vi "OAT Even Time or Speed Segment (XY, 1D Array).vi"(0 "XY signals":cluster{"X":dbl[], "Y":dbl[]}[](array[cluster]) {"X" format="%.2f"; "Y" format="%.2f"}, 1 "x-axis selection":u16(ring)=2 items=["Time", "Revolution", "RPM"], 2 "reset? (F)":bool, 3 "phase input? (F)":bool, 5 "speed profile":T4 {"speed [RPM]" format="%.2f"; "time [s]" format="%.2f"}, 7 "position info":T2, 9 "pulse/revolution (1)":i32=1, 11 "error in (no error)":errorcluster, 12 "segment settings":cluster{"start":dbl, "end":dbl, "step size":dbl} {"step size" format="%.2f"; "end" min=0.0 format="%.2f"; "start" min=0.0 format="%.2f"}, 13 "view info":T1={"dB on? (F)"=FALSE, "unwrap phase? (T)"=TRUE, "unit in degree? (T)"=TRUE}) -> (4 "XY signals out":cluster{"X":dbl[], "Y":dbl[]}[](array[cluster]) {"X" format="%.2f"; "Y" format="%.2f"}, 8 "position info out":T2, 10 "end reached?":bool, 14 "actual segment settings":T3 {"actual step size" format="%.2f"; "actual end" min=0.0 format="%.2f"; "actual start" min=0.0 format="%.2f"}, 15 "error out":errorcluster)   [LabVIEW 2017, in "SoundVib_OAUtility.lvlib"]
doc: "Divides an input signal into even-time segments or even-speed intervals. The input signal of this VI can be an even-angle signal or an XY signal. When you use this VI to divide an XY signal, the XY signal can be only the output of the OAT Order Magnitude and Phase VI or OAT Overall Level Plot VI. Wire data to the <B>even-angle signal</B> input to determine the polymorphic instance to use or manually select the instance."
uses:
  <vilib>/addons/Sound and Vibration/Order Analysis/Utility/SoundVib_OAUtility.lvlib
  <vilib>/addons/Sound and Vibration/Order Analysis/Tach Process/SubVIs/speed profile.ctl
  <vilib>/addons/Sound and Vibration/Order Analysis/Misc/OAT Position Info.ctl
  <vilib>/addons/Sound and Vibration/Order Analysis/Tach Process/SoundVib_TachProcess.lvlib
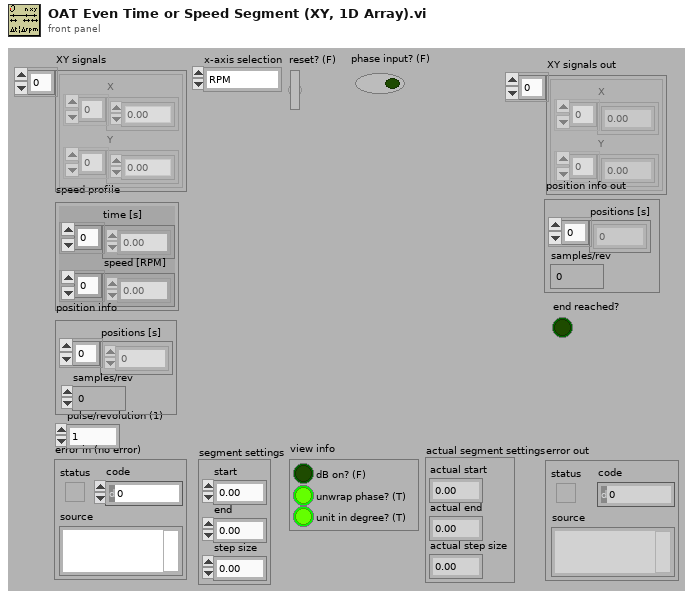
[diagram p1: front panel]
types:
  T1 = cluster{"dB on? (F)":bool, "unwrap phase? (T)":bool, "unit in degree? (T)":bool}
  T2 = typedef "OAT Position Info.ctl" = cluster{"positions [s]":dbl[], "samples/rev":dbl}
  T3 = cluster{"actual start":dbl, "actual end":dbl, "actual step size":dbl}
  T4 = typedef "SoundVib_TachProcess.lvlib/speed profile.ctl" = cluster{"time [s]":dbl[], "speed [RPM]":dbl[]}
  T5 = cluster{"last rev":dbl, "rev indice":dbl[], "time indice":dbl[], "RPM indice":dbl[]}
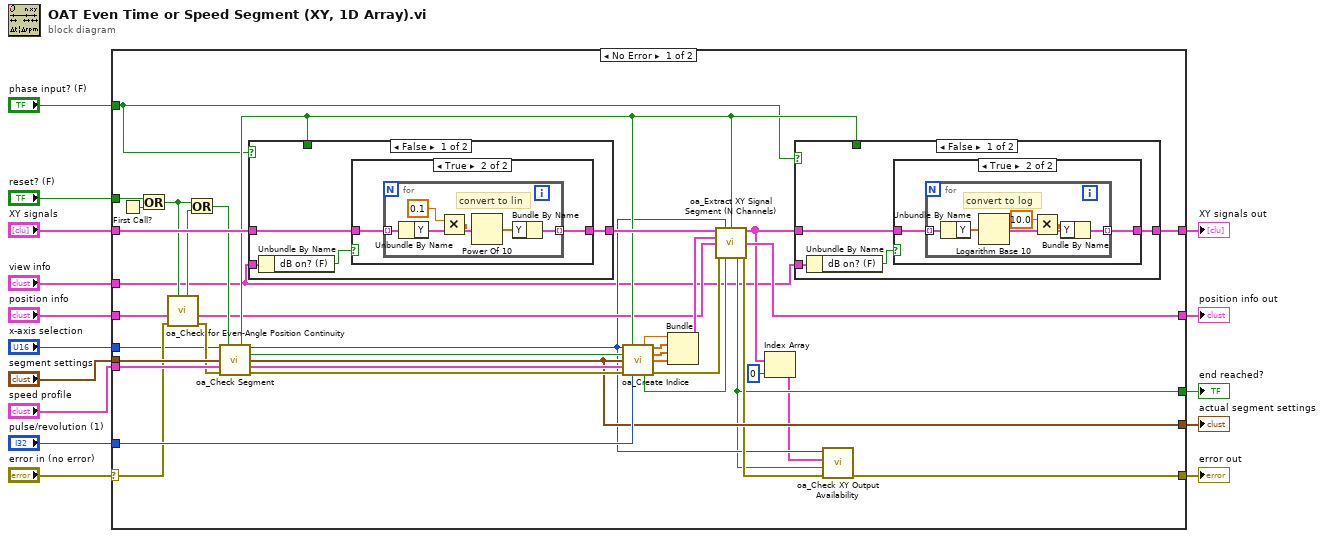
[diagram p0: block diagram]
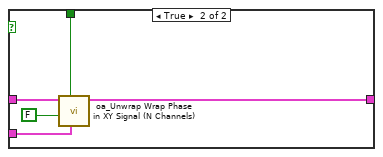
[diagram p3: hidden frame]
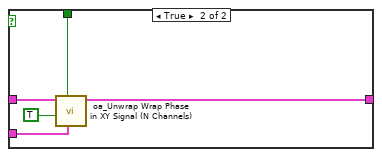
[diagram p5: hidden frame]
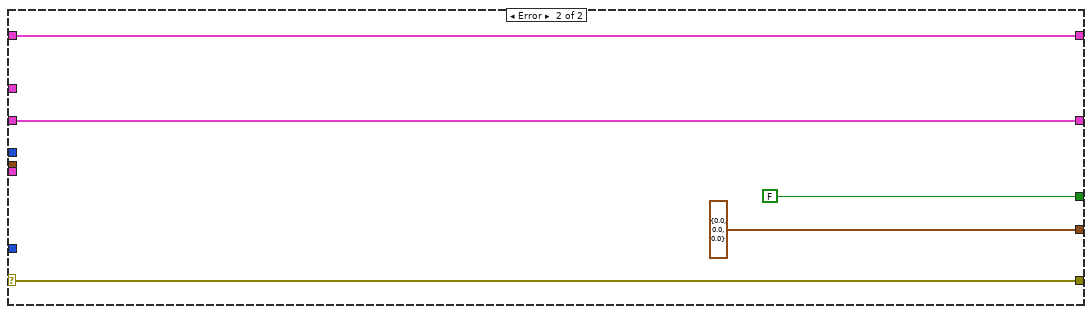
[diagram p6: hidden frame]
diagram:
  n1 = case shown="No Error" "error in (no error)" {
    selector: "error in (no error)" -> [w27 w94]
    tunnel: [w24 w94] -> w1
    tunnel: "reset? (F)" -> [w36 _]
    tunnel: "x-axis selection" -> [w23 _]
    tunnel: "segment settings" -> [w46 _]
    tunnel: "speed profile" -> [w31 _]
    tunnel: [w44 cluster{"start":dbl, "end":dbl, "step":dbl} {"start"=0.0, "end"=0.0, "step"=0.0} ("steps output")] -> w2
    tunnel: "pulse/revolution (1)" -> [w45 _]
    tunnel: "XY signals" -> [w39 w92]
    tunnel: [w21 FALSE ("finish?")] -> w4
    tunnel: "position info" -> [w42 w91]
    tunnel: [w37 w92] -> w5
    tunnel: [w40 w91] -> w3
    tunnel: "phase input? (F)" -> [w17 _]
    tunnel: "view info" -> [w16 _]
    frame No Error {
      n2 = First Call?() -> (First Call?: T/F=w35:bool)
      n3 = Or(x=w36, y=w35) -> (x .or. y?=w29:bool)
      n4 = call <vilib>:"oa_Check for Even-Angle Position Continuity.vi"("reset in"=w29, "error in (no error)"=w27, "even-angle position info"=w42) -> ("error out"=w26:errorcluster, "even-angle position info dup"=w30:T2, "position not continuous"=w28:bool)  [unwired: 6 in]
      n5 = Or(x=w29, y=w28) -> (x .or. y?=w32:bool)
      n6 = call <vilib>:"oa_Check Segment.vi"("X axis selection"=w23, "reset?(F)"=w32, "segment position"=w46, "speed profile"=w31, "error in (no error)"=w26) -> ("reset out"=w33:bool, "X axis selection"=w22:u16, "step found?"=w51:bool, "segment position out"=w44:cluster{"start":dbl, "end":dbl, "step size":dbl}, "dul speed profile"=w52:T4, "error out"=w53:errorcluster)  [unwired: 5 in]
      n7 = case shown="False" w17 {
        tunnel: w39 -> [w73 w89]
        tunnel: [w72 w88] -> w38
        tunnel: w33 -> [_ w87]
        tunnel: w16 -> [w75 w85]
        frame False {
          n8 = Unbundle By Name(w75) -> ("dB on? (F)"=w74:bool)
          n9 = case shown="True" w74 {
            tunnel: w73 -> [w76 w78]
            tunnel: [w76 w77] -> w72
            frame False {
            }
            frame True {
              n10 = for {
                tunnel: w78 -> [w83] mode=indexing
                tunnel: [w82] -> w77 mode=indexing
                # "convert to lin"
                n11 = Unbundle By Name(w83) -> ("Y"=w81:dbl[])
                n12 = Multiply(x=0.1 ("last rev"), y=w81) -> (x*y=w80:dbl[])
                n13 = Power Of 10(x=w80) -> (10^x=w84:dbl[])
                n14 = Bundle By Name(cluster=w83, "Y"=w84) -> (w82:cluster{"X":dbl[], "Y":dbl[]})
              }
            }
          }
        }
        frame True {
          n15 = call <vilib>:"oa_Unwrap Wrap Phase in XY Signal (N Channels).vi"("view"=w85, "reset? (F)"=w87, "Unwrap?"=TRUE, "XY signals"=w89) -> ("XY signals out"=w88:cluster{"X":dbl[], "Y":dbl[]}[])  [unwired: 7 in]
        }
      }
      n16 = call <vilib>:"oa_Create Indice.vi"("X axis selection"=w22, "reset?(F)"=w33, "step found?(F)"=w51, "steps input"=w44, "speed profile"=w52, "error in (no error)"=w53, "pulse/revolution (1)"=w45) -> ("last rev"=w47:dbl, "rev indice"=w48:dbl[], "time indice"=w49:dbl[], "RPM indice"=w50:dbl[], "reach end?"=w34:bool, "error out"=w41:errorcluster)  [unwired: 2 in, 1 out]
      n17 = Bundle("last rev"=w47, "rev indice"=w48, "time indice"=w49, "RPM indice"=w50) -> (w43:T5)  [unwired: 1 in]
      n18 = call <vilib>:"oa_Extract XY Signal Segment (N Channels).vi"("XY signals"=w38, "X axis selection"=w22, "reset? (F)"=w33, "trigger indices"=w43, "position info in"=w30, "error in (no error)"=w41, "indices end?"=w34) -> ("XY signals out"=w20:cluster{"X":dbl[], "Y":dbl[]}[], "position info out"=w40:T2, "reached end?"=w21:bool, "error out"=w25:errorcluster)  [unwired: 5 in]
      n19 = Index Array(array=w20, index=0) -> (element=w19:cluster{"X":dbl[], "Y":dbl[]})
      n20 = case shown="False" w17 {
        tunnel: w20 -> [w55 w71]
        tunnel: [w56 w70] -> w37
        tunnel: w16 -> [w57 w69]
        tunnel: w33 -> [_ w67]
        frame False {
          n21 = Unbundle By Name(w57) -> ("dB on? (F)"=w54:bool)
          n22 = case shown="True" w54 {
            tunnel: w55 -> [w58 w60]
            tunnel: [w58 w59] -> w56
            frame False {
            }
            frame True {
              n23 = for {
                tunnel: w60 -> [w65] mode=indexing
                tunnel: [w64] -> w59 mode=indexing
                # "convert to log"
                n24 = Unbundle By Name(w65) -> ("Y"=w66:dbl[])
                n25 = Logarithm Base 10(1:w66) -> (0:w62:dbl[])
                n26 = Multiply(x=10.0 ("last rev"), y=w62) -> (x*y=w61:dbl[])
                n27 = Bundle By Name(cluster=w65, "Y"=w61) -> (w64:cluster{"X":dbl[], "Y":dbl[]})
              }
            }
          }
        }
        frame True {
          n28 = call <vilib>:"oa_Unwrap Wrap Phase in XY Signal (N Channels).vi"("view"=w69, "reset? (F)"=w67, "Unwrap?"=FALSE, "XY signals"=w71) -> ("XY signals out"=w70:cluster{"X":dbl[], "Y":dbl[]}[])  [unwired: 7 in]
        }
      }
      n29 = call <vilib>:"oa_Check XY Output Availability.vi"("error in (no error)"=w25, "reached end?"=w21, "XY signal"=w19, "x-axis selection"=w22) -> ("error out"=w24:errorcluster)  [unwired: 7 in]
    }
    frame Error {
    }
  }
  "error out" <- w1
  "end reached?" <- w4
  "actual segment settings" <- w2
  "XY signals out" <- w5
  "position info out" <- w3
